vi "Measurement Logic.vi"(8 "error in":errorcluster, 9 "measurement configuration":T2={"Automation Test"=FALSE, "Power sequencing file path"="", "RFmxVNA name"="5842_0", "vCal Name"="VNA-5633", "RFmxVNA Calset Enable"=FALSE, "RFmxVNA Calset Interpolation"=FALSE, "Calset File Path (String)"="", "RFmxVNA attenuation mode"=enum."s2p File", "RFmxVNA Port1 s2p file path (String)"="", "RFmxVNA Port1 s-parameters orientation"=enum."Port2 Towards DUT", "RFmxVNA Port1 Power Compensation"=FALSE, "RFmxVNA Port2 s2p file path (String)"="", "RFmxVNA Port2 s-parameters orientation"=enum."Port1 Towards DUT", "RFmxVNA Port2 Power Compensation"=FALSE, "Port1 Power Level (dBm)"=2.0, "Port1 Test Receiver Attenuation (dB)"=1.2, "Port2 Power Level (dBm)"=2.0, "Port2 Test Receiver Attenuation (dB)"=1.2, "IF Bandwidth (Hz)"=1.0, "Action"=enum."Measure", "Pulse Mode Enabled"=FALSE, "Pulse Period"=0.001, "Pulse Modulator Delay"=0.0, "Pulse Modulator Width"=0.0001, "Pulse Acquisition Auto"=FALSE, "Pulse Acquisition Delay"=2e-05, "Pulse Acquisition Width"=4.665e-05, "Start Frequency (Hz)"=4000000000.0, "Stop Frequency (Hz)"=26000000000.0, "Number of Points"=200, "Measurement S-Parameters"=["S11", "S12", "S21", "S22"], "Phase Trace Type"=0, "Magnitude Units"=0, "SnP File Path (String)"="", "Averaging Enabled"=FALSE, "Averaging Count"=0} {"Magnitude Units" items=["dB", "Linear"]; "Phase Trace Type" items=["Wrapped", "Unwrapped"]; "Stop Frequency (Hz)" format="%.3p"; "Start Frequency (Hz)" format="%.3p"; "Pulse Acquisition Width" format="%.2p"; "Pulse Acquisition Delay" format="%.2p"; "Pulse Modulator Width" format="%.2p"; "Pulse Modulator Delay" format="%.2p"; "Pulse Period" format="%.2p"; "IF Bandwidth (Hz)" format="%.2p"; "Port2 Test Receiver Attenuation (dB)" format="%.2f"; "Port2 Power Level (dBm)" format="%.2f"; "Port1 Test Receiver Attenuation (dB)" format="%.2f"; "Port1 Power Level (dBm)" format="%.2f"}, 10 "measure call context in":refnum<class "Measure Call Context.lvclass">) -> (0 "error out":errorcluster, 1 "measurement results":T1, 2 "measure call context out":refnum<class "Measure Call Context.lvclass">)   [LabVIEW 2023, in "FPT_SParam.lvclass"]
doc: "Contains the core logic for executing the measurement."
uses:
  FPT_SParam.lvclass
  <vilib>/Plug-In SDKs/Measurements/Measure Call Context/Measure Call Context.lvclass
  Measurement Configuration.ctl
  Measurement Results.ctl
  <vilib>/Analysis/baseanly.llb/Mean (DBL).vi
  <extravilib>/ChannelInstances/Event Messenger-bool/Instantiate.vi
  <vilib>/Analysis/NI_AALBase.lvlib
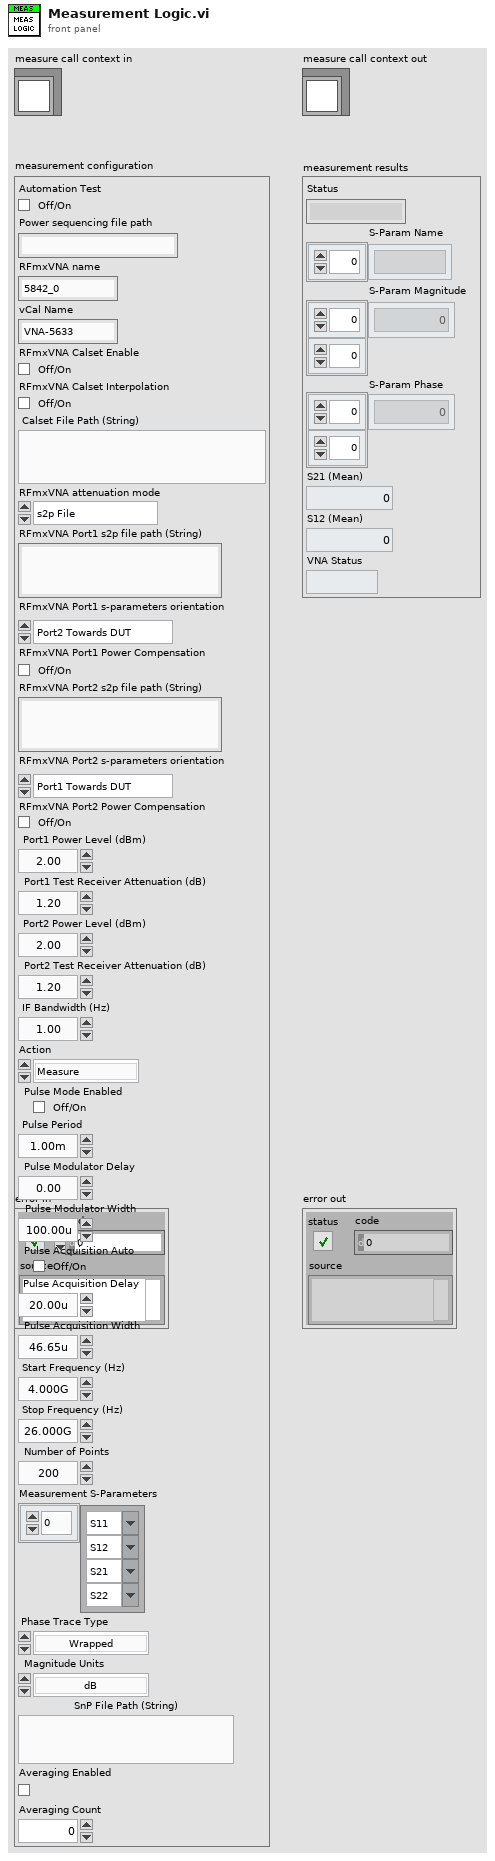
[diagram p1: front panel]
types:
  T1 = typedef "FPT_SParam.lvclass/Measurement Results.ctl" = cluster{"Status":string, "S-Param Name":string[], "S-Param Magnitude":dbl[][], "S-Param Phase":dbl[][], "S21 (Mean)":dbl, "S12 (Mean)":dbl, "VNA Status":string}
  T2 = typedef "FPT_SParam.lvclass/Measurement Configuration.ctl" = cluster{"Automation Test":bool, "Power sequencing file path":string, "RFmxVNA name":string, "vCal Name":string, "RFmxVNA Calset Enable":bool, "RFmxVNA Calset Interpolation":bool, "Calset File Path (String)":string, "RFmxVNA attenuation mode":enum32{"<None>", "s2p File"}, "RFmxVNA Port1 s2p file path (String)":string, "RFmxVNA Port1 s-parameters orientation":enum32{"Port1 Towards DUT", "Port2 Towards DUT"}, "RFmxVNA Port1 Power Compensation":bool, "RFmxVNA Port2 s2p file path (String)":string, "RFmxVNA Port2 s-parameters orientation":enum32{"Port1 Towards DUT", "Port2 Towards DUT"}, "RFmxVNA Port2 Power Compensation":bool, "Port1 Power Level (dBm)":dbl, "Port1 Test Receiver Attenuation (dB)":dbl, "Port2 Power Level (dBm)":dbl, "Port2 Test Receiver Attenuation (dB)":dbl, "IF Bandwidth (Hz)":dbl, "Action":enum32{"Calibrate", "Measure"}, "Pulse Mode Enabled":bool, "Pulse Period":dbl, "Pulse Modulator Delay":dbl, "Pulse Modulator Width":dbl, "Pulse Acquisition Auto":bool, "Pulse Acquisition Delay":dbl, "Pulse Acquisition Width":dbl, "Start Frequency (Hz)":dbl, "Stop Frequency (Hz)":dbl, "Number of Points":i32, "Measurement S-Parameters":string[], "Phase Trace Type":i32, "Magnitude Units":i32, "SnP File Path (String)":string, "Averaging Enabled":bool, "Averaging Count":u32}
  T3 = cluster{"measurement configuration":T2, "measurement results":T1}
  T4 = enum32{"Power On Dut", "Switching", "De-embedding + Measurement", "Power Off Dut"}[]
  T5 = typedef "RFmxVNA Config - SParam.ctl" = cluster{"Resource Name":refnum<k15>, "vCal Name":string, "RFmxVNA Calset Enable":bool, "RFmxVNA Calset Interpolation":bool, "Calset File Path":string, "RFmxVNA attenuation mode":enum32{"<None>", "s2p File"}, "RFmxVNA Port1 s2p file path":string, "RFmxVNA Port1 s-parameters orientation":enum32{"Port1 Towards DUT", "Port2 Towards DUT"}, "RFmxVNA Port1 Power Compensation":bool, "RFmxVNA Port2 s2p file path":string, "RFmxVNA Port2 s-parameters orientation":enum32{"Port1 Towards DUT", "Port2 Towards DUT"}, "RFmxVNA Port2 Power Compensation":bool, "Port1 Power Level (dBm)":dbl, "Port1 Test Receiver Attenuation (dB)":dbl, "Port2 Power Level (dBm)":dbl, "Port2 Test Receiver Attenuation (dB)":dbl, "IF Bandwidth (Hz)":dbl, "Frequency Sweep":cluster{"Start Frequency (Hz)":dbl, "Stop Frequency (Hz)":dbl, "Number of Points":i32}}
  T6 = typedef "Test Config - SParam.ctl" = cluster{"Action":enum16{"Calibrate", "Measure"}, "Pulse Mode":cluster{"Pulse Mode Enabled":bool, "Pulse Period (s)":dbl, "Pulse Modulator Delay (s)":dbl, "Pulse Modulator Width (s)":dbl, "Pulse Acquisition Auto":bool, "Pulse Acquisition Delay (s)":dbl, "Pulse Acquisition Width (s)":dbl}, "Frequency Sweep":cluster{"Start Frequency (Hz)":dbl, "Stop Frequency (Hz)":dbl, "Number of Points":i32}, "S-Parameters":string[], "Magnitude Units":i32, "Phase Trace Type":i32, "SnP File Path":string, "Averaging Enabled":bool, "Averaging Count":u32}
  T7 = typedef "Event Messenger-bool.lvlib/))Channel.ctl" = refnum<queue>
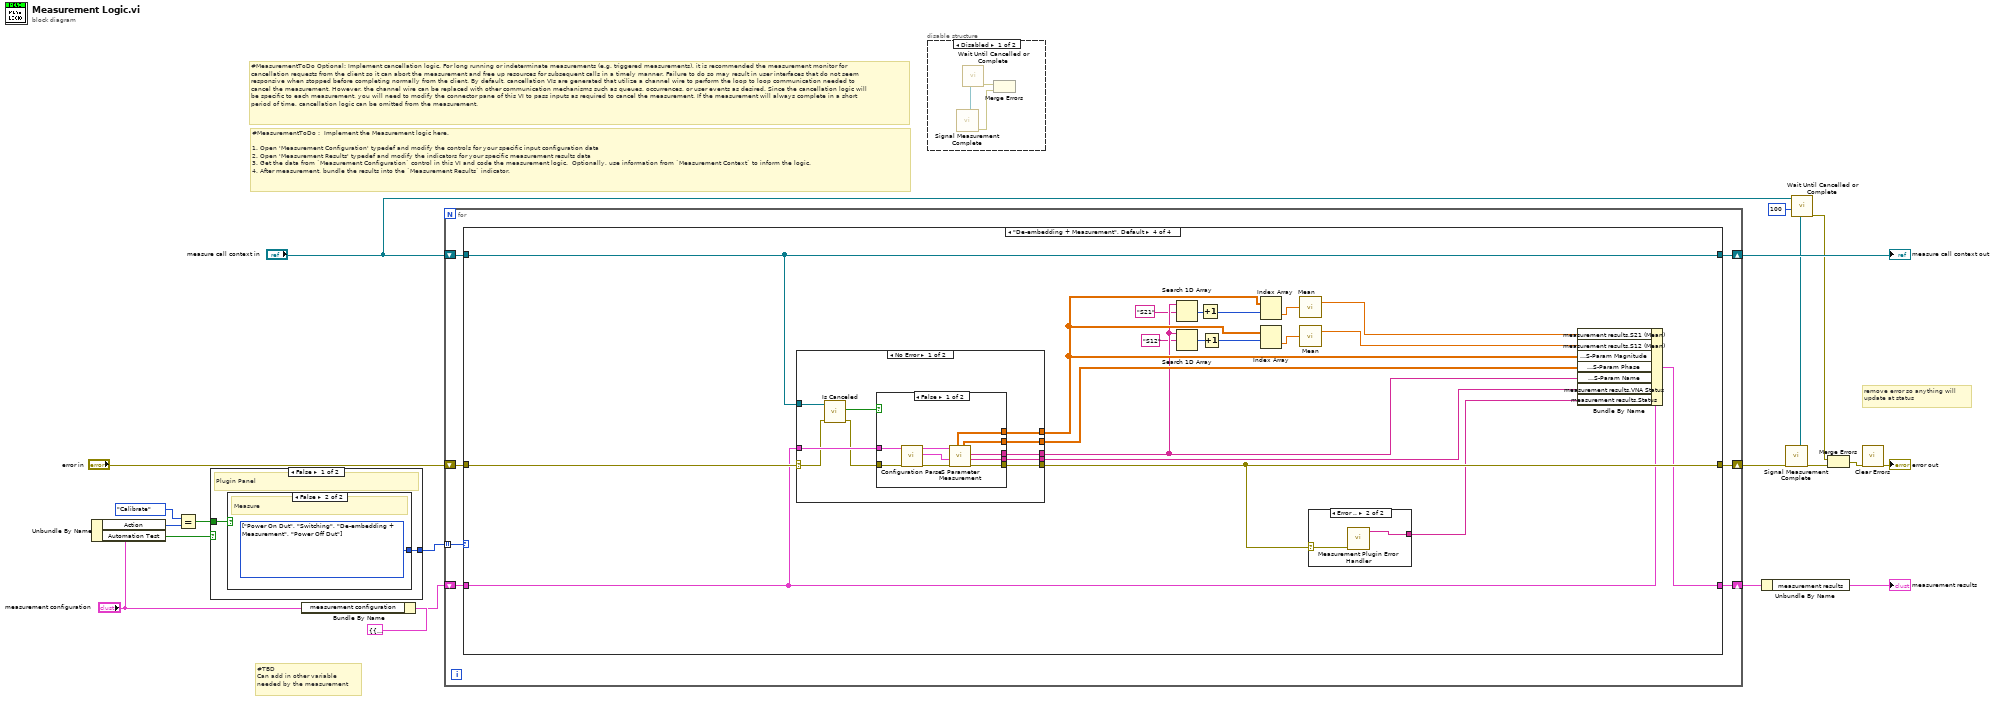
[diagram p0: block diagram]
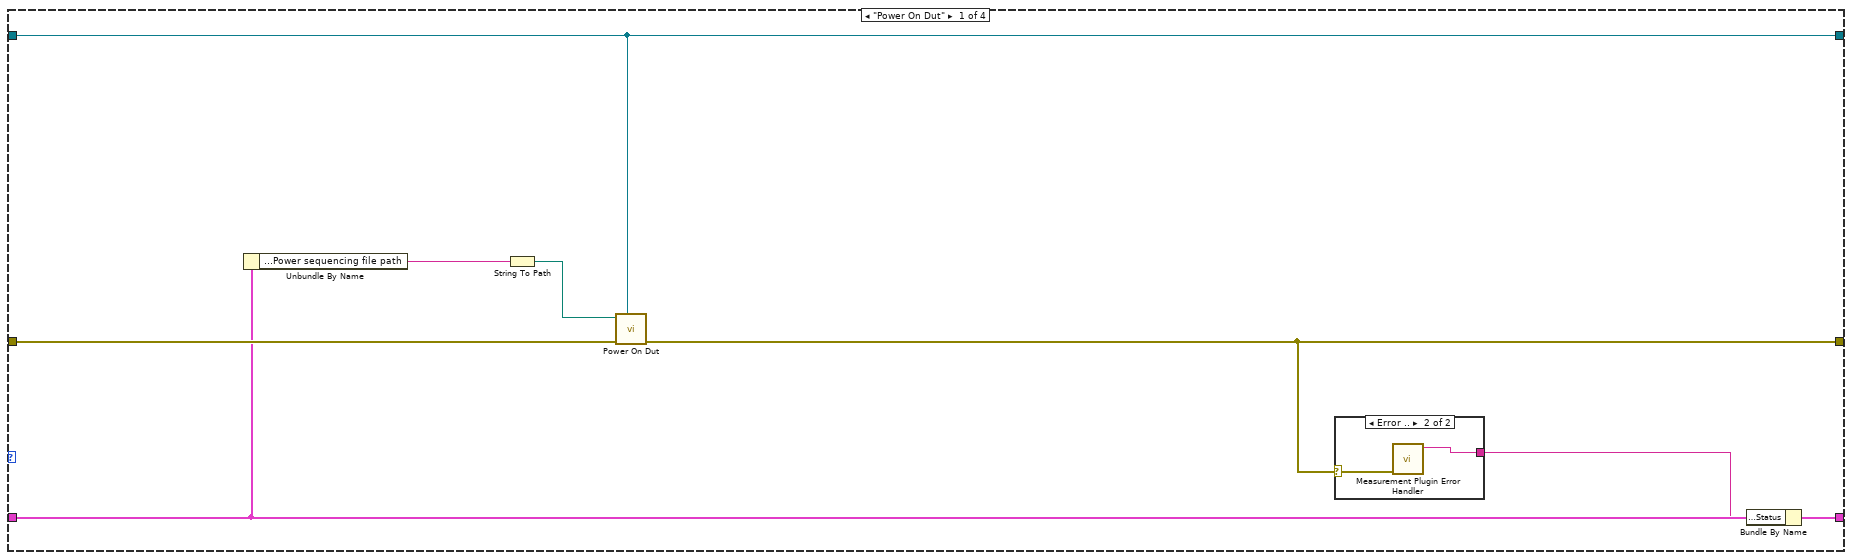
[diagram p2: hidden frame]
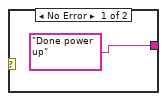
[diagram p3: hidden frame]
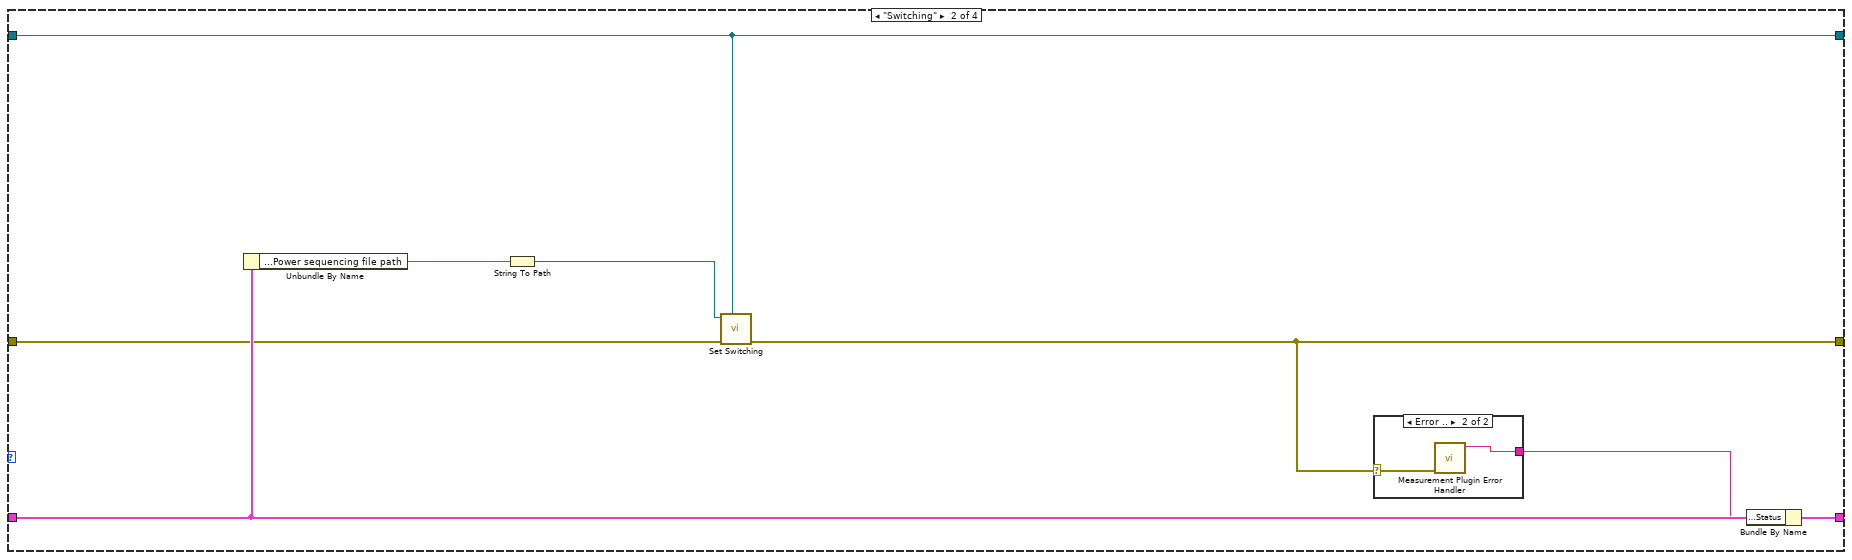
[diagram p4: hidden frame]
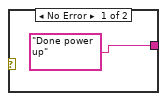
[diagram p5: hidden frame]
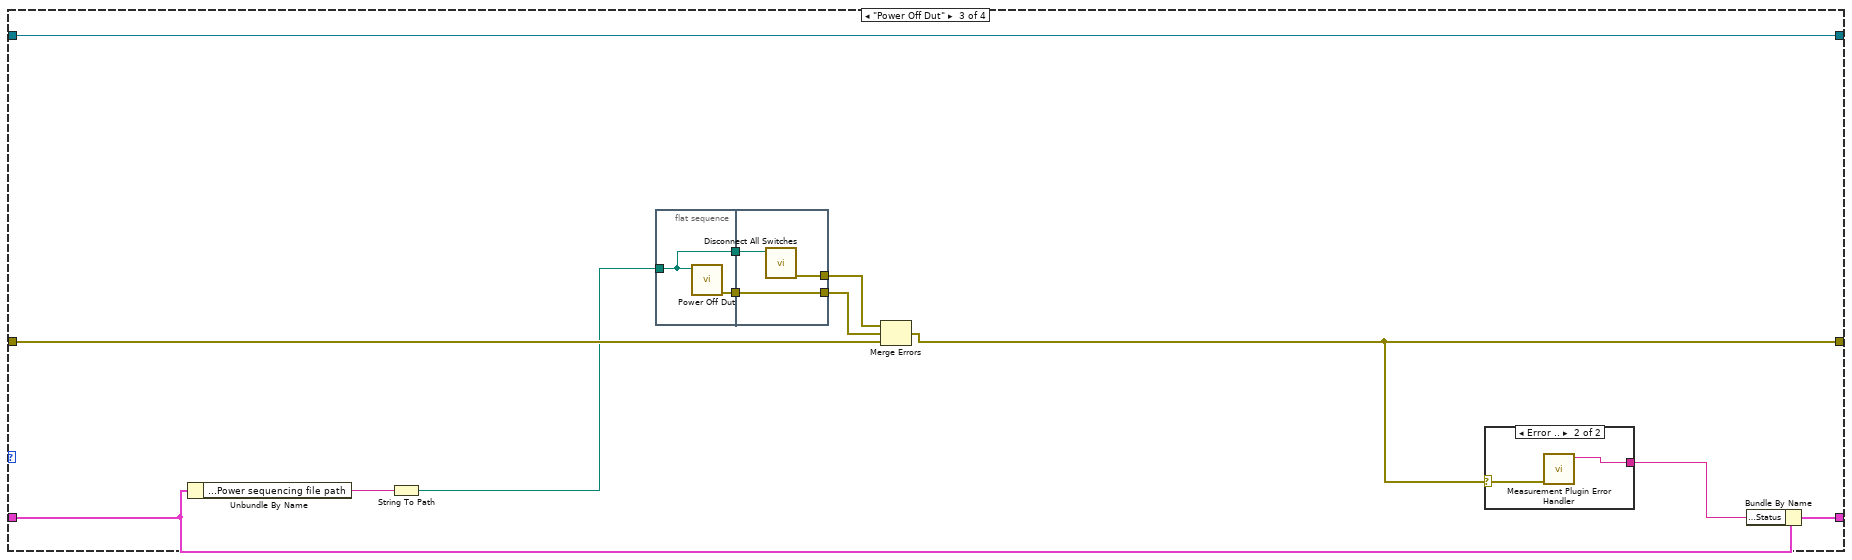
[diagram p6: hidden frame]
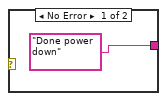
[diagram p7: hidden frame]
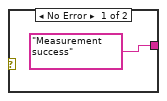
[diagram p8: hidden frame]
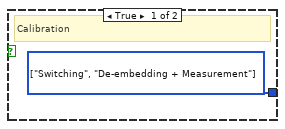
[diagram p12: hidden frame]
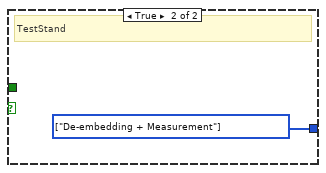
[diagram p13: hidden frame]
diagram:
  # "remove error so anything will\nupdate at status"
  # "#TBD\nCan add in other variable\nneeded by the measurement"
  # "#MeasurementToDo Optional: Implement cancellation logic. For long running or indeterminate measurements (e.g. triggered measurements), it is recommended the measurement monitor for cancellation requests from the client so it can abort the measurement and free up resources for subsequent calls in a timely manner. Failure to do so may result in user interfaces that do not seem responsive when stopped before completing normally from the client. By default, cancellation VIs are generated that utilize a channel wire to perform the loop to loop communication needed to cancel the measurement. However, the channel wire can be replaced with other communication mechanisms such as queues, occurrences, or user events as desired. Since the cancellation logic will be specific to each measurement, you will need to modify the connector pane of this VI to pass inputs as required to cancel the measurement. If the measurement will always complete in a short period of time, cancellation logic can be omitted from the measurement."
  # "#MeasurementToDo :  Implement the Measurement logic here.\n\n1. Open 'Measurement Configuration' typedef and modify the controls for your specific input configuration data\n2. Open 'Measurement Results' typedef and modify the indicators for your specific measurement results data\n3. Get the data from `Measurement Configuration` control in this VI and code the measurement logic.  Optionally, use information from `Measurement Context` to inform the logic.\n4. After measurement, bundle the results into the `Measurement Results` indicator."
  n1 = Unbundle By Name("measurement configuration") -> ("Action"=w12:enum32{"Calibrate", "Measure"}, "Automation Test"=w9:bool)
  n2 = Equal?(x=enum32{"Calibrate", "Measure"}."Calibrate", y=w12) -> (x = y?=w8:bool)
  n3 = case shown="False" w9 {
    tunnel: [w22 w25] -> w10
    tunnel: w8 -> [w21 _]
    frame False {
      # "Plugin Panel"
      n4 = case shown="False" w21 {
        tunnel: [w23 w24] -> w22
        frame True {
          w23 = T4 [enum."Switching", enum."De-embedding + Measurement"] items=["Power On Dut", "Switching", "De-embedding + Measurement", "Power Off Dut"]
          # "Calibration"
        }
        frame False {
          w24 = T4 [enum."Power On Dut", enum."Switching", enum."De-embedding + Measurement", enum."Power Off Dut"] items=["Power On Dut", "Switching", "De-embedding + Measurement", "Power Off Dut"]
          # "Measure"
        }
      }
    }
    frame True {
      w25 = T4 [enum."De-embedding + Measurement"] items=["Power On Dut", "Switching", "De-embedding + Measurement", "Power Off Dut"]
      # "TestStand"
    }
  }
  n5 = Bundle By Name(cluster=T3 {"measurement configuration"={"Automation Test"=FALSE, "Power sequencing file path"="", "RFmxVNA name"="5842_0", "vCal Name"="VNA-5633", "RFmxVNA Calset Enable"=FALSE, "RFmxVNA Calset Interpolation"=FALSE, "Calset File Path (String)"="", "RFmxVNA attenuation mode"=enum."s2p File", "RFmxVNA Port1 s2p file path (String)"="", "RFmxVNA Port1 s-parameters orientation"=enum."Port2 Towards DUT", "RFmxVNA Port1 Power Compensation"=FALSE, "RFmxVNA Port2 s2p file path (String)"="", "RFmxVNA Port2 s-parameters orientation"=enum."Port1 Towards DUT", "RFmxVNA Port2 Power Compensation"=FALSE, "Port1 Power Level (dBm)"=2.0, "Port1 Test Receiver Attenuation (dB)"=1.2, "Port2 Power Level (dBm)"=2.0, "Port2 Test Receiver Attenuation (dB)"=1.2, "IF Bandwidth (Hz)"=1.0, "Action"=enum."Measure", "Pulse Mode Enabled"=FALSE, "Pulse Period"=0.001, "Pulse Modulator Delay"=0.0, "Pulse Modulator Width"=0.0001, "Pulse Acquisition Auto"=FALSE, "Pulse Acquisition Delay"=2e-05, "Pulse Acquisition Width"=4.665e-05, "Start Frequency (Hz)"=4000000000.0, "Stop Frequency (Hz)"=26000000000.0, "Number of Points"=200, "Measurement S-Parameters"=["S11", "S12", "S21", "S22"], "Phase Trace Type"=0, "Magnitude Units"=0, "SnP File Path (String)"="", "Averaging Enabled"=FALSE, "Averaging Count"=0}, "measurement results"={"Status"="", "S-Param Name"=[], "S-Param Magnitude"=[], "S-Param Phase"=[], "S21 (Mean)"=0.0, "S12 (Mean)"=0.0, "VNA Status"=""}}, "measurement configuration"="measurement configuration") -> (w18:T3)
  n6 = for {
    tunnel: w10 -> [w31] mode=indexing
    shift-right: [w26] -> w4
    shift-left: "error in" -> [w32]
    shift-right: [w27] -> w16
    shift-left: w18 -> [w30]
    shift-right: [w28] -> w17
    shift-left: "measure call context in" -> [w29]
    n7 = case shown="\"De-embedding + Measurement\", Default" w31 {
      tunnel: w32 -> [w40 w45 w61 w89]
      tunnel: w30 -> [w39 w51 w62 w88]
      tunnel: w29 -> [w33 w44 w65 w75]
      tunnel: [w34 w47 w60 w94] -> w26
      tunnel: [w33 w44 w65 w75] -> w28
      tunnel: [w37 w49 w63 w92] -> w27
      frame "Power On Dut" {
        n8 = Unbundle By Name(w39) -> ("measurement configuration.Power sequencing file path"=w36:string)
        n9 = String To Path(string=w36) -> (path=w35:path)
        n10 = call "Power On Dut.vi"("measure call context in"=w33, "error in"=w40, "Power sequencing file path"=w35) -> ("error out"=w34:errorcluster)  [unwired: 7 in, 1 out]
        n11 = case shown="Error .." w34 {
          selector: w34 -> [_ w43]
          tunnel: ["Done power up" w42] -> w38
          frame No Error {
          }
          frame Error {
            n12 = call "Measurement Plugin Error Handler.vi"("error in"=w43) -> ("Status Message (Error)"=w42:string)  [unwired: 9 in, 1 out]
          }
        }
        n13 = Bundle By Name(cluster=w39, "measurement results.Status"=w38) -> (w37:T3)
      }
      frame "Switching" {
        n14 = Unbundle By Name(w51) -> ("measurement configuration.Power sequencing file path"=w48:string)
        n15 = String To Path(string=w48) -> (path=w46:path)
        n16 = call "Set Switching.vi"("measure call context in"=w44, "error in"=w45, "File Path"=w46) -> ("error out"=w47:errorcluster)  [unwired: 7 in, 1 out]
        n17 = case shown="Error .." w47 {
          selector: w47 -> [_ w54]
          tunnel: ["Done power up" w53] -> w50
          frame No Error {
          }
          frame Error {
            n18 = call "Measurement Plugin Error Handler.vi"("error in"=w54) -> ("Status Message (Error)"=w53:string)  [unwired: 9 in, 1 out]
          }
        }
        n19 = Bundle By Name(cluster=w51, "measurement results.Status"=w50) -> (w49:T3)
      }
      frame "Power Off Dut" {
        n20 = Unbundle By Name(w62) -> ("measurement configuration.Power sequencing file path"=w66:string)
        n21 = String To Path(string=w66) -> (path=w57:path)
        n22 = flat-sequence {
          tunnel: w57 -> [w70]
          tunnel: [w71] -> w59
          tunnel: [w70] -> w58
          tunnel: [w74] -> w56
          tunnel: w59 -> [w74]
          tunnel: [w73] -> w55
          tunnel: w58 -> [w72]
          frame #0 {
            n23 = call "Power Off Dut.vi"("Power Sequencing File Path"=w70) -> ("error out"=w71:errorcluster)  [unwired: 10 in]
          }
          frame #1 {
            n24 = call "Disconnect All Switches.vi"("File Path"=w72) -> ("error out"=w73:errorcluster)  [unwired: 10 in]
          }
        }
        n25 = Merge Errors(w55, w56, w61) -> (w60:errorcluster)
        n26 = case shown="Error .." w60 {
          selector: w60 -> [_ w69]
          tunnel: ["Done power down" w68] -> w64
          frame No Error {
          }
          frame Error {
            n27 = call "Measurement Plugin Error Handler.vi"("error in"=w69) -> ("Status Message (Error)"=w68:string)  [unwired: 9 in, 1 out]
          }
        }
        n28 = Bundle By Name(cluster=w62, "measurement results.Status"=w64) -> (w63:T3)
      }
      frame "De-embedding + Measurement", Default {
        n29 = case shown="No Error" w89 {
          selector: w89 -> [w101 w119]
          tunnel: [w107 w119] -> w94
          tunnel: [w106 _] -> w83
          tunnel: [w105 _] -> w91
          tunnel: [w104 _] -> w90
          tunnel: [w103 _] -> w82
          tunnel: w88 -> [w102 _]
          tunnel: w75 -> [w98 _]
          frame No Error {
            n30 = call <vilib>:"Is Canceled.vi"("error in"=w101, "measure call context in"=w98) -> ("error out"=w100:errorcluster, "is canceled?"=w99:bool)  [unwired: 7 in, 1 out]
            n31 = case shown="False" w99 {
              tunnel: [w117 w118] -> w107
              tunnel: [w113 _] -> w106
              tunnel: [w112 _] -> w105
              tunnel: [w111 _] -> w104
              tunnel: [w110 _] -> w103
              tunnel: w102 -> [w109 _]
              tunnel: w100 -> [w108 w118]
              frame False {
                n32 = call "Configuration Parse.vi"("error in"=w108, "UI Controls"=w109) -> ("error out"=w115:errorcluster, "RFmxVNA Settings"=w116:T5, "Test Configuration"=w114:T6)  [unwired: 7 in]
                n33 = call "S Parameter Measurement.vi"("error in"=w115, "RFmxVNA Settings"=w116, "Test Configuration"=w114) -> ("error out"=w117:errorcluster, "VNA Status"=w111:string, "S-Param Name"=w110:string[], "S-Param Phase"=w112:dbl[][], "S-Param Magnitude"=w113:dbl[][])  [unwired: 3 in, 1 out]
              }
              frame True {
              }
            }
          }
          frame Error {
          }
        }
        n34 = Search 1D Array(1D array=w82, element="S21") -> (index of element=w79:i32)  [unwired: 1 in]
        n35 = Search 1D Array(1D array=w82, element="S12") -> (index of element=w77:i32)  [unwired: 1 in]
        n36 = Increment(x=w79) -> (x+1=w78:i32)
        n37 = Increment(x=w77) -> (x+1=w76:i32)
        n38 = Index Array(array=w83, index (row)=w78) -> (element=w87:dbl[])  [unwired: 1 in]
        n39 = Index Array(array=w83, index (row)=w76) -> (element=w85:dbl[])  [unwired: 1 in]
        n40 = call-poly <vilib>:"Mean.vi"("X"=w87) -> ("mean"=w86:dbl)  [unwired: 1 out]
        n41 = call-poly <vilib>:"Mean.vi"("X"=w85) -> ("mean"=w84:dbl)  [unwired: 1 out]
        n42 = case shown="Error .." w94 {
          selector: w94 -> [_ w97]
          tunnel: ["Measurement success" w96] -> w93
          frame No Error {
          }
          frame Error {
            n43 = call "Measurement Plugin Error Handler.vi"("error in"=w97) -> ("Status Message (Error)"=w96:string)  [unwired: 9 in, 1 out]
          }
        }
        n44 = Bundle By Name(cluster=w88, "measurement results.S21 (Mean)"=w86, "measurement results.S12 (Mean)"=w84, "measurement results.S-Param Magnitude"=w83, "measurement results.S-Param Phase"=w91, "measurement results.S-Param Name"=w82, "measurement results.VNA Status"=w90, "measurement results.Status"=w93) -> (w92:T3)
      }
    }
  }
  "measure call context out" <- w17
  n45 = disable-structure shown="Disabled" {
    frame Disabled {
      n46 = call "Signal Measurement Complete.vi"() -> ("error out"=w121:errorcluster, "done channel"=w122:T7)  [unwired: 10 in]
      n47 = call "Wait Until Cancelled or Complete.vi"("done channel"=w122) -> ("error out"=w120:errorcluster)  [unwired: 9 in, 1 out]
      n48 = Merge Errors(w120, w121) -> ()  [unwired: 1 out]
    }
    frame Enabled {
    }
  }
  n49 = Unbundle By Name(w16) -> ("measurement results"=→"measurement results":T1)
  n50 = call "Signal Measurement Complete.vi"("error in (no error)"=w4) -> ("error out"=w3:errorcluster, "done channel"=w2:T7)  [unwired: 9 in]
  n51 = call "Wait Until Cancelled or Complete.vi"("done channel"=w2, "ms polling interval"=100, "measure call context in"="measure call context in") -> ("error out"=w6:errorcluster)  [unwired: 7 in, 1 out]
  n52 = Merge Errors(w6, w3) -> (w7:errorcluster)
  n53 = call <vilib>:"Clear Errors.vi"("error in (no error)"=w7) -> ("error out"=→"error out":errorcluster)  [unwired: 5 in, 1 out]
